vi "Add and Map Paired Outputs.vi"(8 "error in (no error)":errorcluster, 9 "Paired Module Output Channels":refnum<class "TBM channel.lvclass">[](array[class]), 10 "engine configuration in":refnum<class "engine configuration.lvclass">, 11 "E2E configuration in":refnum<class "E2E Tag Exchange configuration.lvclass">) -> (0 "error out":errorcluster, 2 "engine configuration out":refnum<class "engine configuration.lvclass">, 3 "E2E configuration out":refnum<class "E2E Tag Exchange configuration.lvclass">)   [LabVIEW 2015, in "E2E Tag Exchange editor node.lvclass"]
uses:
  E2E Tag Exchange editor node.lvclass
  <vilib>/NI/Tag Bus Module Framework/channel/TBM channel.lvclass
  <vilib>/NI/Module Execution Interface/Engine Configuration/engine configuration.lvclass
  module/configuration/E2E Tag Exchange configuration.lvclass
  module/configuration/E2E Tag Exchange configuration.lvclass/E2E Tag Exchange configuration.ctl
  <vilib>/NI/Tag Bus Module Framework/channel/channel classification.ctl
  <vilib>/NI/Tag Bus/tag/tag descriptor.lvclass/tag descriptor.ctl
  <vilib>/NI/Tag Bus Module Framework/channel/TBM channel.lvclass/TBM channel.ctl
  <vilib>/NI/Configuration Framework/serializable configuration/NISE_CEF_serializable configuration.lvclass/NISE_CEF_serializable configuration.ctl
  <vilib>/Utility/LVClass/Get LV Class Name.vi
  <vilib>/NI/Configuration Framework/error generator/NISE_error generator.vi
  <vilib>/NI/Configuration Framework/serializable configuration/NISE_CEF_serializable configuration.lvclass
  <vilib>/NI/Tag Bus/tag/tag descriptor.lvclass
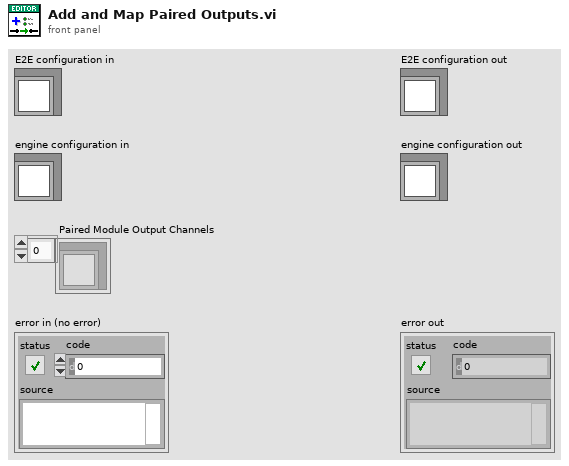
[diagram p1: front panel]
types:
  T1 = typedef "TBM channel.lvclass/channel classification.ctl" = enum16{"input data", "output data", "processing parameter", "processing result"}
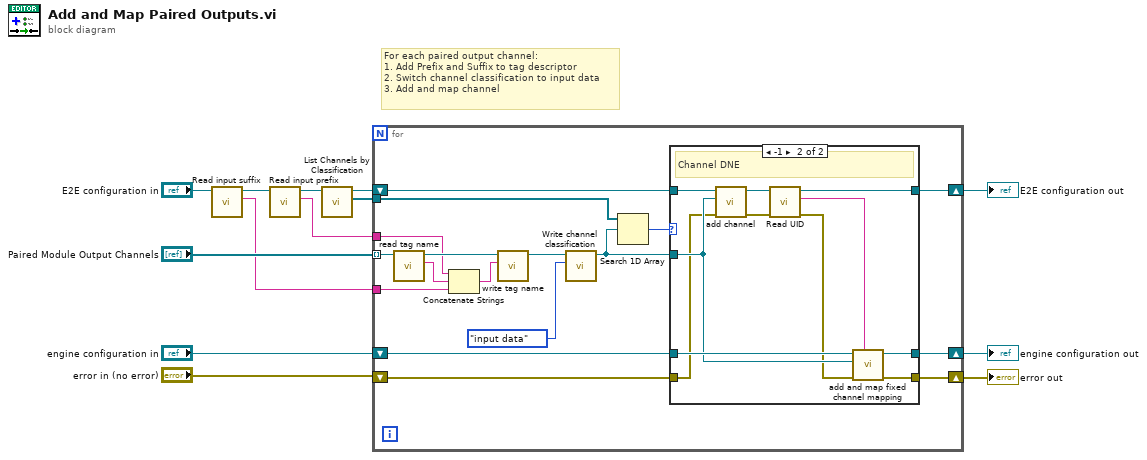
[diagram p0: block diagram]
diagram:
  # "For each paired output channel:\n1. Add Prefix and Suffix to tag descriptor\n2. Switch channel classification to input data\n3. Add and map channel"
  n1 = call "Read input suffix.vi"("E2E Tag Exchange configuration in"="E2E configuration in") -> ("input suffix"=w4:string, "E2E Tag Exchange configuration out"=w3:refnum<class "E2E Tag Exchange configuration.lvclass">)  [unwired: 8 in, 1 out]
  n2 = call "Read input prefix.vi"("E2E Tag Exchange configuration in"=w3) -> ("input prefix"=w1:string, "E2E Tag Exchange configuration out"=w2:refnum<class "E2E Tag Exchange configuration.lvclass">)  [unwired: 8 in, 1 out]
  n3 = call "List Channels by Classification.vi"("E2E configuration in"=w2) -> ("Input Channels"=w11:refnum<class "TBM channel.lvclass">[], "E2E configuration out"=w12:refnum<class "E2E Tag Exchange configuration.lvclass">)  [unwired: 8 in, 1 out]
  n4 = for {
    tunnel: "Paired Module Output Channels" -> [w20] mode=indexing
    tunnel: w11 -> [w29]
    shift-right: [w23] -> w7
    shift-left: "engine configuration in" -> [w26]
    shift-right: [w24] -> w6
    shift-left: w12 -> [w27]
    shift-right: [w22] -> w8
    shift-left: "error in (no error)" -> [w21]
    tunnel: w4 -> [w18]
    tunnel: w1 -> [w14]
    n5 = call <vilib>:"read tag name.vi"("system tag in"=w20) -> ("name"=w16:string, "system tag out"=w17:refnum<class "TBM channel.lvclass">)  [unwired: 8 in, 1 out]
    n6 = Concatenate Strings(w14, w16, w18) -> (w15:string)
    n7 = call <vilib>:"write tag name.vi"("name"=w15, "system tag in"=w17) -> ("system tag out"=w19:refnum<class "TBM channel.lvclass">)  [unwired: 8 in, 1 out]
    n8 = call <vilib>:"Write channel classification.vi"("channel classification"=channel_classification."input data", "channel in"=w19) -> ("channel out"=w25:refnum<class "TBM channel.lvclass">)  [unwired: 8 in, 1 out]
    n9 = Search 1D Array(1D array=w29, element=w25) -> (index of element=w28:i32)  [unwired: 1 in]
    n10 = case shown="-1" w28 {
      tunnel: w27 -> [w32 w44]
      tunnel: w26 -> [w31 w43]
      tunnel: w25 -> [_ w42]
      tunnel: [w32 w37] -> w24
      tunnel: [w31 w36] -> w23
      tunnel: [w33 w35] -> w22
      tunnel: w21 -> [w33 w34]
      frame Default {
        # "Channel Exists"
      }
      frame -1 {
        # "Channel DNE"
        n11 = call "add channel.vi"("error in (no error)"=w34, "channel"=w42, "E2E configuration in"=w44) -> ("error out"=w40:errorcluster, "E2E configuration out"=w41:refnum<class "E2E Tag Exchange configuration.lvclass">)  [unwired: 7 in]
        n12 = call <vilib>:"Read UID.vi"("error in"=w40, "configuration in"=w41) -> ("error out"=w38:errorcluster, "instance id"=w39:string, "configuration out"=w37:refnum<class "E2E Tag Exchange configuration.lvclass">)  [unwired: 7 in]
        n13 = call <vilib>:"add and map fixed channel mapping.vi"("module instance"=w39, "error in"=w38, "fixed channel"=w42, "engine configuration in"=w43) -> ("error out"=w35:errorcluster, "engine configuration out"=w36:refnum<class "engine configuration.lvclass">)  [unwired: 6 in]
      }
    }
  }
  "E2E configuration out" <- w6
  "engine configuration out" <- w7
  "error out" <- w8
